vi "Name.vi"(8 "error in (no error)":errorcluster, 11 "Player in":refnum<class "Player.lvclass">) -> (0 "error out":errorcluster, 2 "Name":string, 3 "Player out":refnum<class "Player.lvclass">)   [LabVIEW 2020, in "Reversi.lvlib" / "Player.lvclass"]
uses:
  Player.lvclass
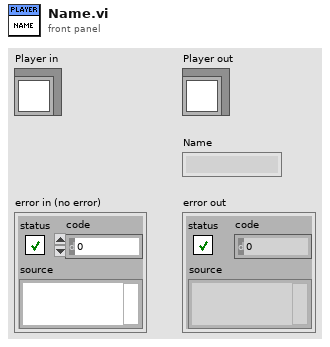
[diagram p1: front panel]
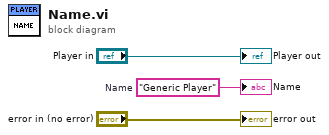
[diagram p0: block diagram]
diagram:
  w1 = "Generic Player"  # Name
  "error out" <- "error in (no error)"
  "Player out" <- "Player in"
  "Name" <- w1
